vi "writeMCSBatch.vi"(7 "Current Param Value":dbl, 9 "Raw Data Folder":path, 10 "File Name":string, 11 "Full Scan Name":string) -> (0 "error out":errorcluster)   [LabVIEW 2015]
panel:
  out "concatenated string":string
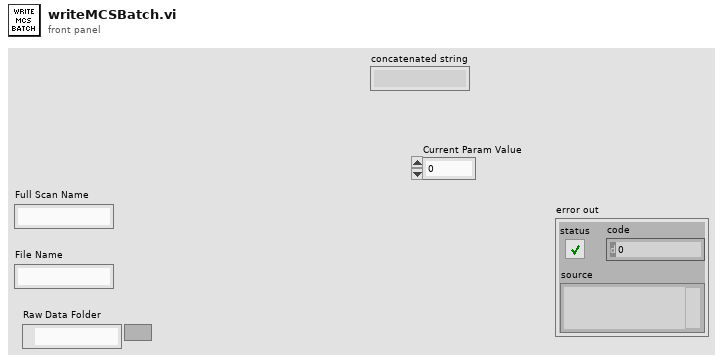
[diagram p1: front panel]
types:
  T1 = enum16{"open", "replace", "create", "open or create", "replace or create", "replace or create with confirmation"}
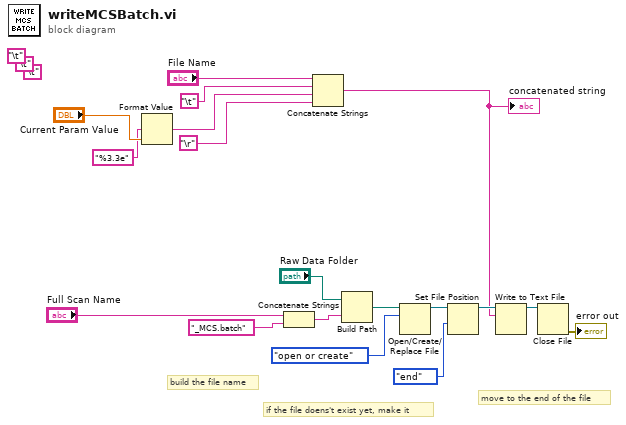
[diagram p0: block diagram]
diagram:
  (unwired) "\t"
  (unwired) "\t"
  (unwired) "\t"
  # "move to the end of the file"
  # "if the file doens't exist yet, make it"
  # "build the file name"
  n1 = Format Value(format string="%3.3e", value (0)="Current Param Value") -> (output string=w3:string)  [unwired: 1 in]
  n2 = Concatenate Strings("Full Scan Name", "_MCS.batch" ("string")) -> (w17:string)
  n3 = Concatenate Strings("File Name", "\t", w3, "\r") -> (w7:string)
  "concatenated string" <- w7
  n4 = Build Path(base path="Raw Data Folder", name or relative path=w17) -> (appended path=w15:path)
  n5 = Open/Create/Replace File(file path (use dialog)=w15, operation (0:open)=T1."open or create") -> (refnum out=w11:refnum<file>)  [unwired: 4 in, 2 out]
  n6 = Set File Position(refnum=w11, from (0:start)=enum16{"start", "end", "current"}."end") -> (refnum out=w12:refnum<file>)  [unwired: 2 in, 1 out]
  n7 = Write to Text File(file (use dialog)=w12, text=w7) -> (refnum out=w13:refnum<file>)  [unwired: 2 in, 2 out]
  n8 = Close File(refnum=w13) -> (error out=→"error out":errorcluster)  [unwired: 1 in, 1 out]
